vi "temp_probe_calibrator.vi"() -> ()   [LabVIEW 2010]
uses:
  <vilib>/Instr/_visa.llb/VISA Configure Serial Port (Instr).vi
  <vilib>/Utility/file.llb/Write To Spreadsheet File (string).vi
  <vilib>/Analysis/NI_AALBase.lvlib
  <vilib>/Analysis/NI_AALPro.lvlib
panel:
  out "estimatedTemps":dbl[](array[numeric]) format="%.3g"
  out "XY Graph":T1(graph)
  in  "Path":path=path "C:/Users/OA-user/Documents/OAlab/data"
  in  "fileName":string="tempProbe_cal_data_"
  out "CalOutput":string[][](array[string])
  in  "RefText":string="fluke_1523_#1085081"
  in  "headers":string[](array[string])=["location", "probeType", "channel", "Ohm->Temp", "date", "reference"]
  in  "labels":string[][](array[string])=[["cell", "TJ36-44004-1/8"], ["acidBottle", "TJ36-44004-1/8"], ["burrette1", "SA1-TH-44004-40-T"], ["burrette2", "SA1-TH-44004-40-T"], ["room", "unknown"]]
  out "currentSet":dbl format="%.3g"
  out "currentPoint":i32=20
  out "numPoints":i32=20
  out "rawOhmsAll":dbl[][](array[numeric])
  out "flukeTempsAll":dbl[](array[numeric]) format="%.3g"
  out "FlukeTempAvg":dbl format="%.3g"
  in  "chillTemps":dbl[](array[numeric])
  out "Waveform Chart":dbl(graph)
  out "currentTime":timestamp format="%<%X>T"
  out "lastRead":timestamp format="%<%X>T"
  in  "nextRead":timestamp format="%<%X>T"
  in  "Neslab Port IN":refnum<visa-resource-name>="COM12"
  in  "minutes@temp":dbl=20.0
  out "rawOhm":dbl[](array[numeric])
  out "FlukeTemp":dbl format="%.3g"
  in  "stop":bool
  in  "Agilent Settings":T2={"Agilent COM Port"="", "Probe Channels (csv)"="103,104,105,106,107", "Number of Readings"=10}
  in  "Fluke Settings":T3={"COM Port"="COM13", "Baud Rate"=9600, "Data Bit"=8, "Parity"=0, "Bytes to Read"=7}
  out "error out":errorcluster
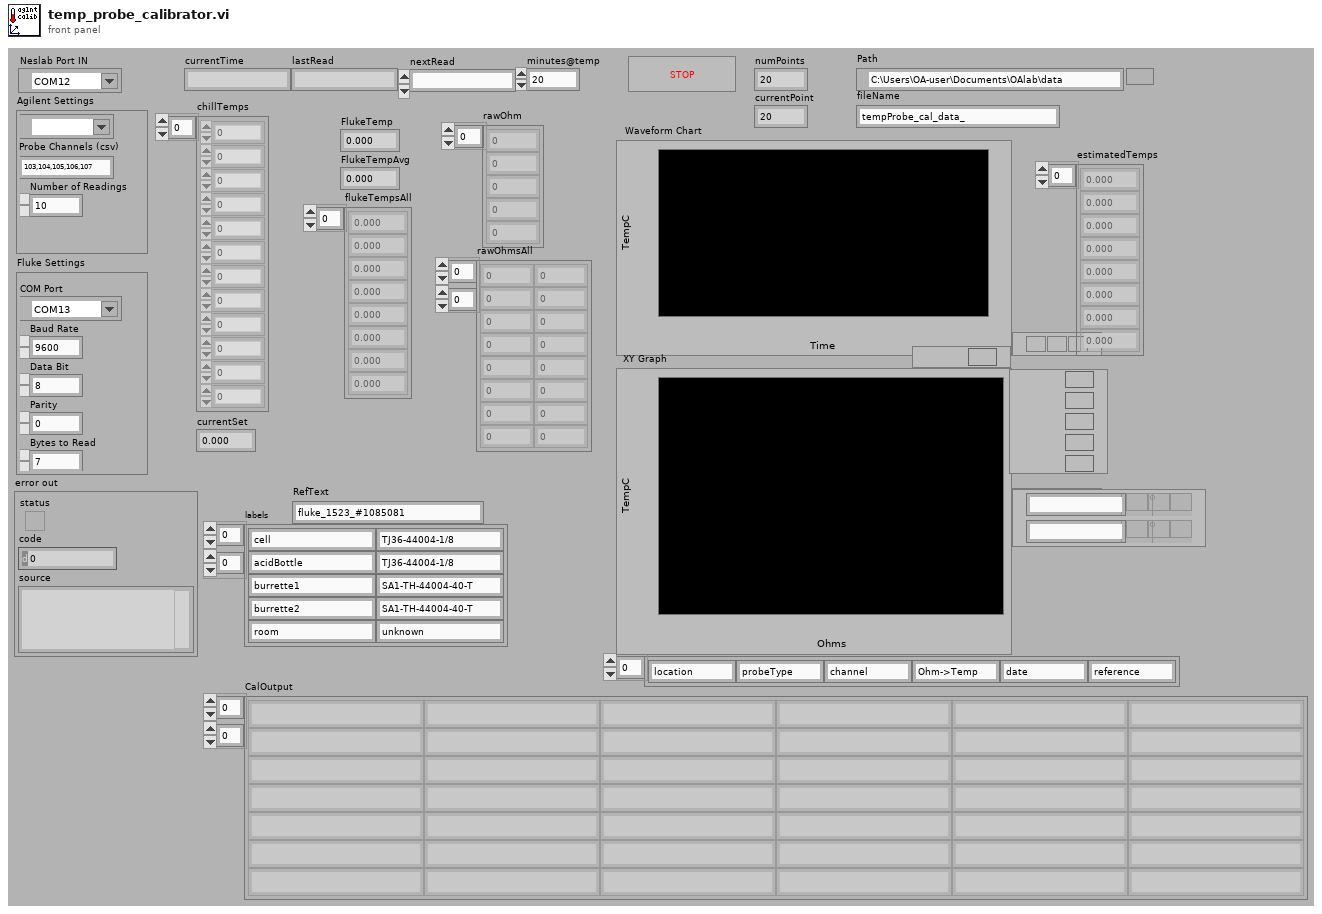
[diagram p1: front panel]
types:
  T1 = cluster{"flukeTempsAll":dbl[], "rawOhmsAll":dbl[]}[]
  T2 = cluster{"Agilent COM Port":refnum<visa-resource-name>, "Probe Channels (csv)":string, "Number of Readings":i32}
  T3 = cluster{"COM Port":refnum<visa-resource-name>, "Baud Rate":u32, "Data Bit":i8, "Parity":i8, "Bytes to Read":u32}
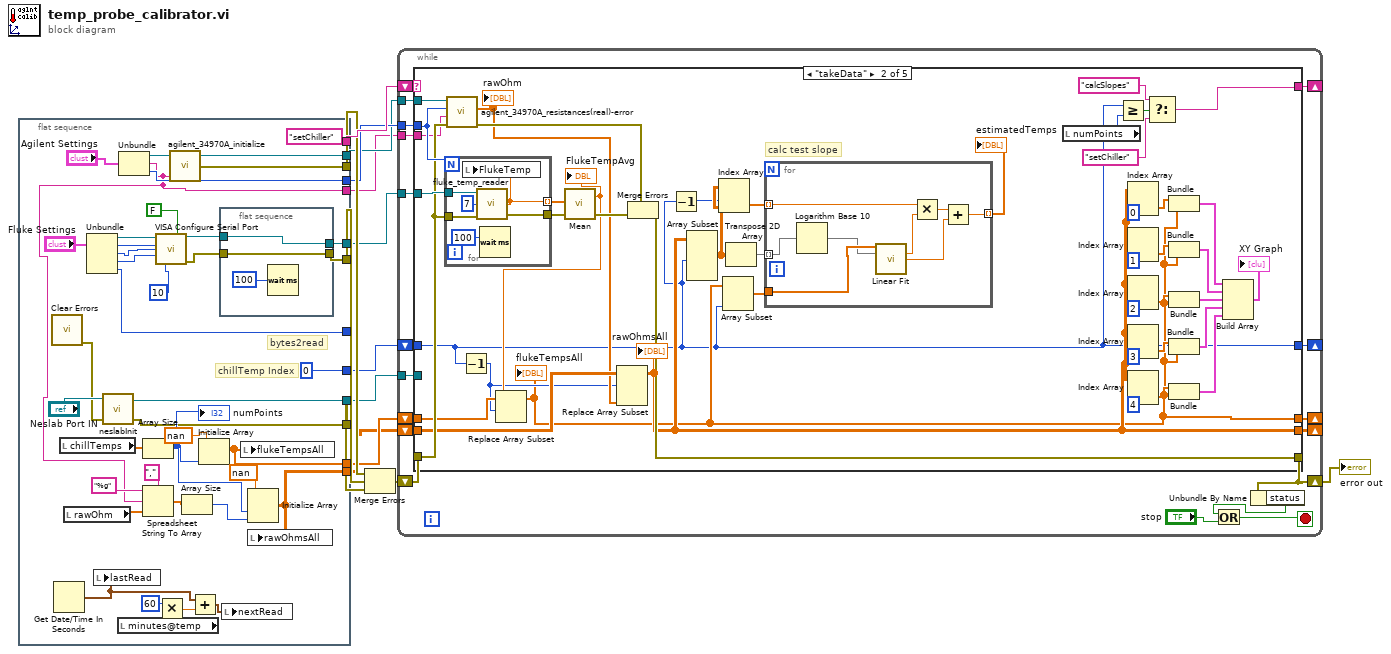
[diagram p0: block diagram]
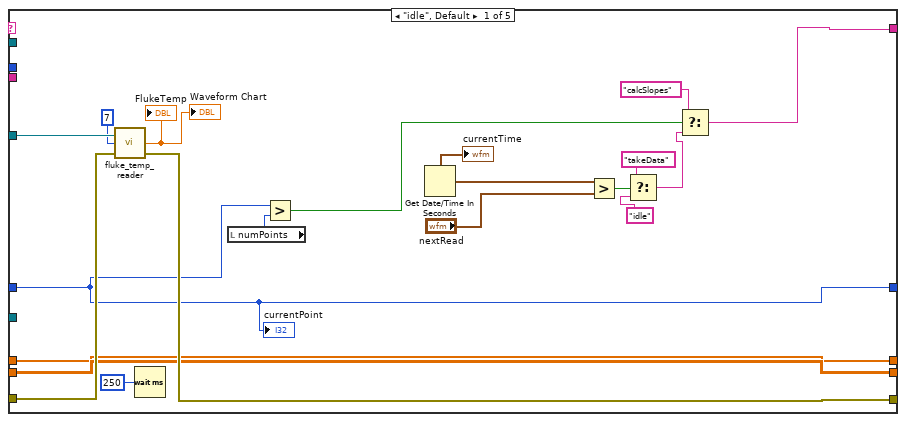
[diagram p2: hidden frame]
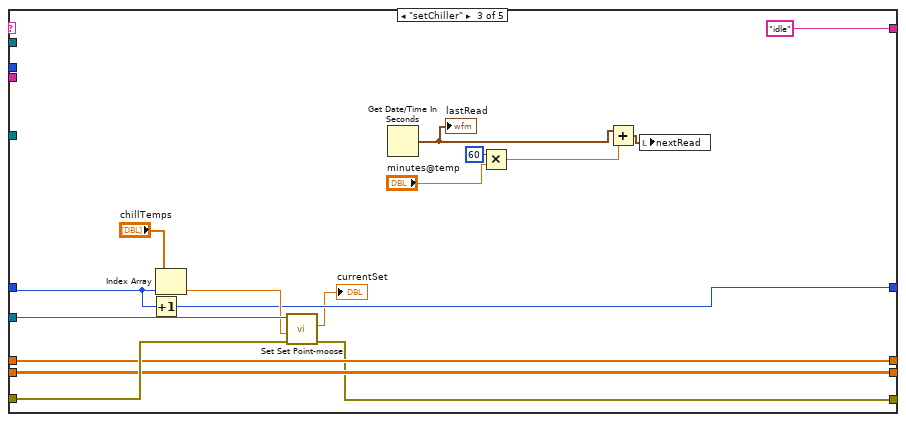
[diagram p3: hidden frame]
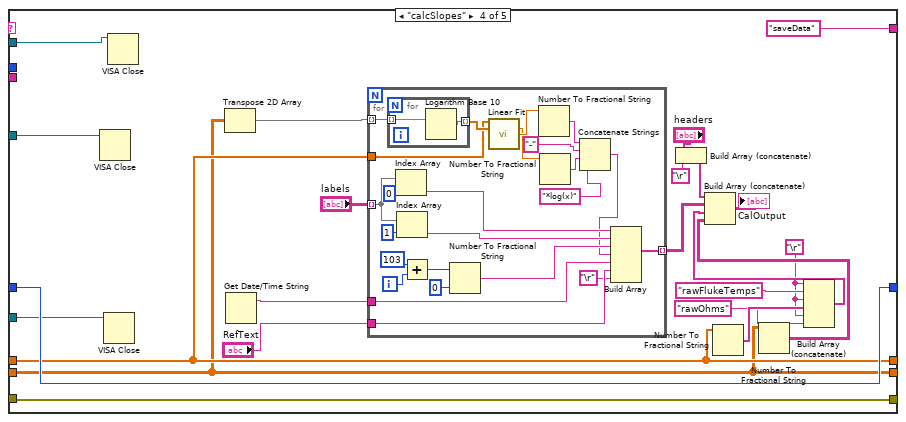
[diagram p4: hidden frame]
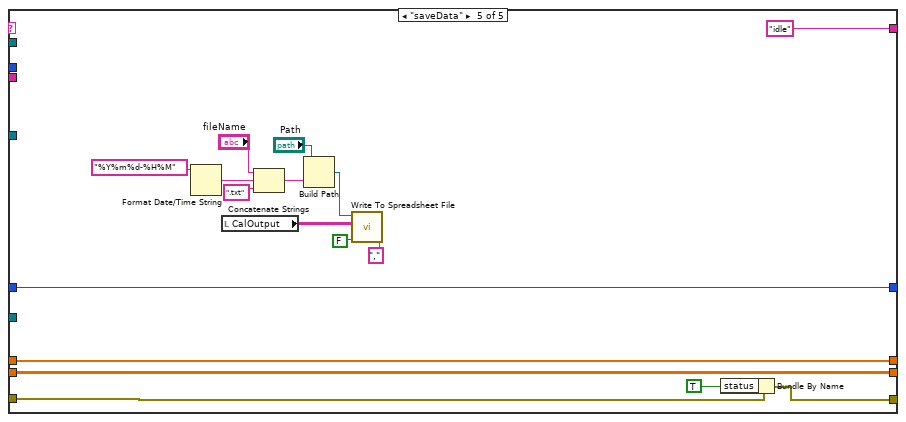
[diagram p5: hidden frame]
diagram:
  n1 = flat-sequence {
    tunnel: [w52] -> w9
    tunnel: [w50] -> w12
    tunnel: [w48] -> w5
    tunnel: [w47] -> w13
    tunnel: [w41] -> _
    tunnel: [w38] -> w6
    tunnel: [w30] -> w1
    tunnel: [w16] -> w11
    tunnel: ["setChiller"] -> w14
    tunnel: [w17] -> w8
    tunnel: [0] -> w7
    tunnel: [w24] -> w4
    tunnel: [w23] -> w3
    frame #0 {
      # "chillTemp Index"
      # "bytes2read"
      n2 = call <vilib>:"Clear Errors.vi"() -> ("error out"=w15:errorcluster)  [unwired: 7 in]
      n3 = Get Date/Time In Seconds() -> (seconds since 1Jan1904=w36:timestamp)
      n4 = local read "chillTemps"() -> (w29:dbl[])
      n5 = local read "rawOhm"() -> (w26:dbl[])
      n6 = Unbundle("Fluke Settings") -> ("COM Port"=w45:refnum<visa-resource-name>, "Baud Rate"=w44:u32, "Data Bit"=w43:i8, "Parity"=w42:i8, "Bytes to Read"=w41:u32)
      n7 = local write "lastRead"(w36) -> ()
      n8 = call "neslabInit.vi"("error in (no error)"=w15, "COM Port"="Neslab Port IN") -> ("error out"=w16:errorcluster, "COM Port Out"=w17:refnum<visa-resource-name>)  [unwired: 1 in, 1 out]
      n9 = local read "minutes@temp"() -> (w19:dbl)
      n10 = Unbundle("Agilent Settings") -> ("Agilent COM Port"=w39:refnum<visa-resource-name>, "Probe Channels (csv)"=w30:string, "Number of Readings"=w38:i32)
      n11 = Array Size(array=w29) -> (size(s)=w22:i32)
      "numPoints" <- w22
      n12 = Spreadsheet String To Array(delimiter (Tab)=",", format string="%g", spreadsheet string=w30, array type (2D Dbl)=w26) -> (array=w33:dbl[])
      n13 = call-poly "VISA Configure Serial Port"("VISA resource name"=w45, "Enable Termination\nChar (T)"=FALSE, "baud rate (9600)"=w44, "data bits (8)"=w43, "parity (0:none)"=w42, "stop bits (10: 1 bit)"=10) -> ("VISA resource name out"=w51:refnum<visa-resource-name>, "error out"=w49:errorcluster)  [unwired: 8 in]
      n14 = Multiply(x=60, y=w19) -> (x*y=w20:dbl)
      n15 = call "agilent_34970A_initialize.vi"("resistance channels (csv)"=w30, "Agilent 34970A Port"=w39) -> ("34970A Error Out"=w47:errorcluster, "34970A Port Out"=w48:refnum<visa-resource-name>)  [unwired: 1 in, 1 out]
      n16 = Array Size(array=w33) -> (size(s)=w25:i32)
      n17 = Add(x=w36, y=w20) -> (x+y=w35:timestamp)
      n18 = Initialize Array(nan ("FlukeTempAvg"), w22) -> (w24:dbl[])
      n19 = flat-sequence {
        tunnel: [w56] -> w52
        tunnel: w51 -> [w56]
        tunnel: [w55] -> w50
        tunnel: w49 -> [w55]
        frame #0 {
          n20 = Wait (ms)(milliseconds to wait=100) -> ()  [unwired: 1 out]
        }
      }
      n21 = local write "nextRead"(w35) -> ()
      n22 = local write "flukeTempsAll"(w24) -> ()
      n23 = Initialize Array(nan ("FlukeTempAvg"), w22, w25) -> (w23:dbl[][])
      n24 = local write "rawOhmsAll"(w23) -> ()
    }
  }
  n25 = Merge Errors(w13, w12, w11) -> (w10:errorcluster)
  n26 = while {
    shift-right: [w60] -> w2
    shift-left: w10 -> [w74]
    tunnel: w9 -> [w73]
    tunnel: w8 -> [w72]
    shift-right: [w70] -> _
    shift-left: w7 -> [w71]
    shift-right: [w69] -> _
    shift-left: w14 -> [w75]
    tunnel: w6 -> [w68]
    tunnel: w5 -> [w67]
    shift-right: [w64] -> _
    shift-left: w4 -> [w66]
    shift-right: [w63] -> _
    shift-left: w3 -> [w65]
    tunnel: w1 -> [w58]
    stop <- w61 stop-if-true
    n27 = case shown="\"takeData\"" w75 {
      tunnel: w74 -> [w93 w134 w167 w189 w220]
      tunnel: w73 -> [w92 w137 _ w186 _]
      tunnel: w72 -> [_ _ w168 w187 _]
      tunnel: w71 -> [w76 w95 w164 w190 w231]
      tunnel: [w76 w95 w156 w190 w231] -> w70
      tunnel: [w88 w127 w154 w189 w219] -> w60
      tunnel: [w78 w121 "idle" "saveData" "idle"] -> w69
      tunnel: w68 -> [_ w136 _ _ _]
      tunnel: w67 -> [_ w138 _ w188 _]
      tunnel: w66 -> [w86 w130 w160 w178 w232]
      tunnel: w65 -> [w87 w129 w161 w175 w233]
      tunnel: [w86 w97 w160 w178 w232] -> w64
      tunnel: [w87 w106 w161 w175 w233] -> w63
      tunnel: w58 -> [_ w126 _ _ _]
      frame "idle", Default {
        n28 = call "fluke_temp_reader.vi"("error in (no error)"=w93, "Bytes to Read"=7, "COM Port In"=w92) -> ("error out"=w88:errorcluster, "Temp"=→"FlukeTemp" →"Waveform Chart":dbl)  [unwired: 1 out]
        n29 = Wait (ms)(milliseconds to wait=250) -> ()  [unwired: 1 out]
        n30 = local read "numPoints"() -> (w82:i32)
        n31 = Greater?(x=w76, y=w82) -> (0:w80:bool)
        n32 = Get Date/Time In Seconds() -> (seconds since 1Jan1904=w90:timestamp)
        "currentTime" <- w90
        n33 = Greater?(x=w90, y="nextRead") -> (0:w84:bool)
        n34 = Select(t="takeData", s=w84, f="idle") -> (s? t:f=w81:string)
        n35 = Select(t="calcSlopes", s=w80, f=w81) -> (s? t:f=w78:string)
        "currentPoint" <- w76
      }
      frame "takeData" {
        # "calc test slope"
        n36 = for {
          N: w136 -> [_]
          tunnel: w137 -> [w152]
          tunnel: w134 -> [w151]
          tunnel: [w150] -> w135 mode=indexing
          tunnel: [w149] -> w133
          n37 = call "fluke_temp_reader.vi"("error in (no error)"=w151, "Bytes to Read"=7, "COM Port In"=w152) -> ("error out"=w149:errorcluster, "Temp"=w150:dbl)  [unwired: 1 out]
          n38 = local write "FlukeTemp"(w150) -> ()
          n39 = Wait (ms)(milliseconds to wait=100) -> ()  [unwired: 1 out]
        }
        n40 = call "agilent_34970A_resistances(real)-error.vi"("error in (no error)"=w134, "Channels"=w126, "Readings"=w136, "Agilent Port In"=w138) -> ("error out"=w132:errorcluster, "Resistances"=w128:dbl[])  [unwired: 2 out]
        "rawOhm" <- w128
        n41 = Decrement(x=w95) -> (x-1=w109:i32)
        n42 = call <vilib>:"Mean.vi"("X"=w135) -> ("mean"=w131:dbl)  [unwired: 1 out]
        "FlukeTempAvg" <- w131
        n43 = Replace Array Subset(array=w130, new element=w131, index=w109) -> (w97:dbl[])
        "flukeTempsAll" <- w97
        n44 = Replace Array Subset(array=w129, new element=w128, index (row)=w109) -> (w106:dbl[][])  [unwired: 1 in]
        "rawOhmsAll" <- w106
        n45 = Merge Errors(w132, w133) -> (w127:errorcluster)
        n46 = Decrement(x=w95) -> (x-1=w96:i32)
        n47 = Array Subset(array=w106, length (row)=w95) -> (w104:dbl[][])  [unwired: 3 in]
        n48 = Index Array(array=w104, index (row)=w96) -> (element=w103:dbl[])  [unwired: 1 in]
        n49 = Array Subset(array=w97, length=w95) -> (w107:dbl[])  [unwired: 1 in]
        n50 = Transpose 2D Array(2D array=w104) -> (transposed array=w108:dbl[][])
        n51 = for {
          tunnel: w108 -> [w142] mode=indexing
          tunnel: w107 -> [w141]
          tunnel: [w143] -> w105 mode=indexing
          tunnel: w103 -> [w139] mode=indexing
          n52 = Logarithm Base 10(1:w142) -> (0:w140:dbl[])
          n53 = call <vilib>:"Linear Fit.vi"("Y"=w141, "X"=w140) -> ("slope"=w146:dbl, "intercept"=w144:dbl)  [unwired: 9 in, 3 out]
          n54 = Multiply(x=w139, y=w146) -> (x*y=w145:dbl)
          n55 = Add(x=w145, y=w144) -> (x+y=w143:dbl)
        }
        "estimatedTemps" <- w105
        n56 = local read "numPoints"() -> (w125:i32)
        n57 = Greater Or Equal?(x=w95, y=w125) -> (x >= y?=w124:bool)
        n58 = Index Array(array=w106, index (col)=0) -> (element=w102:dbl[])  [unwired: 1 in]
        n59 = Index Array(array=w106, index (col)=1) -> (element=w101:dbl[])  [unwired: 1 in]
        n60 = Index Array(array=w106, index (col)=2) -> (element=w100:dbl[])  [unwired: 1 in]
        n61 = Index Array(array=w106, index (col)=3) -> (element=w99:dbl[])  [unwired: 1 in]
        n62 = Index Array(array=w106, index (col)=4) -> (element=w98:dbl[])  [unwired: 1 in]
        n63 = Select(t="calcSlopes", s=w124, f="setChiller") -> (s? t:f=w121:string)
        n64 = Bundle(w102, w97) -> (w115:cluster{dbl[], dbl[]})  [unwired: 1 in]
        n65 = Bundle(w101, w97) -> (w113:cluster{dbl[], dbl[]})  [unwired: 1 in]
        n66 = Bundle(w100, w97) -> (w114:cluster{dbl[], dbl[]})  [unwired: 1 in]
        n67 = Bundle(w99, w97) -> (w112:cluster{dbl[], dbl[]})  [unwired: 1 in]
        n68 = Bundle(w98, w97) -> (w111:cluster{dbl[], dbl[]})  [unwired: 1 in]
        n69 = Build Array(w115, w113, w114, w112, w111) -> (→"XY Graph":cluster{dbl[], dbl[]}[])
      }
      frame "setChiller" {
        n70 = Increment(x=w164) -> (x+1=w156:i32)
        n71 = Index Array(array="chillTemps", index=w164) -> (element=w165:dbl)
        n72 = call "Set Set Point-moose.vi"("COM Port IN"=w168, "Numerical\nSet Value"=w165, "error in\n(no error)"=w167) -> ("Numeric\nReading Value"=→"currentSet":dbl, "error out"=w154:errorcluster)  [unwired: 3 in, 2 out]
        n73 = Get Date/Time In Seconds() -> (seconds since 1Jan1904=w159:timestamp)
        "lastRead" <- w159
        n74 = Multiply(x=60, y="minutes@temp") -> (x*y=w157:dbl)
        n75 = Add(x=w159, y=w157) -> (x+y=w162:timestamp)
        n76 = local write "nextRead"(w162) -> ()
      }
      frame "calcSlopes" {
        w172 = "\r"
        n77 = VISA Close(VISA resource name=w186) -> ()  [unwired: 1 in, 1 out]
        n78 = VISA Close(VISA resource name=w187) -> ()  [unwired: 1 in, 1 out]
        n79 = VISA Close(VISA resource name=w188) -> ()  [unwired: 1 in, 1 out]
        n80 = Transpose 2D Array(2D array=w175) -> (transposed array=w185:dbl[][])
        n81 = Get Date/Time String() -> (date string=w183:string)  [unwired: 3 in, 1 out]
        n82 = for {
          tunnel: w185 -> [w215] mode=indexing
          tunnel: w178 -> [w194]
          tunnel: "labels" -> [w213] mode=indexing
          tunnel: w183 -> [w203]
          tunnel: "RefText" -> [w202]
          tunnel: [w201] -> w181 mode=indexing
          i -> [w211]
          n83 = for {
            tunnel: w215 -> [w217] mode=indexing
            tunnel: [w216] -> w195 mode=indexing
            n84 = Logarithm Base 10(1:w217) -> (0:w216:dbl)
          }
          n85 = Index Array(array=w213, index=0) -> (element=w207:string)
          n86 = Index Array(array=w213, index=1) -> (element=w206:string)
          n87 = Add(x=103, y=w211) -> (x+y=w209:i32)
          n88 = Number To Fractional String(number=w209, precision (6)=0) -> (F-format string=w205:string)  [unwired: 2 in]
          n89 = call <vilib>:"Linear Fit.vi"("Y"=w194, "X"=w195) -> ("slope"=w192:dbl, "intercept"=w193:dbl)  [unwired: 9 in, 3 out]
          n90 = Number To Fractional String(number=w193) -> (F-format string=w208:string)  [unwired: 3 in]
          n91 = Number To Fractional String(number=w192) -> (F-format string=w199:string)  [unwired: 3 in]
          n92 = Concatenate Strings(w208, "-", w199, "*log(x)") -> (w204:string)
          n93 = Build Array(w207, w206, w205, w204, w203, w202, "\r") -> (w201:string[])
        }
        n94 = Build Array (concatenate)("headers", "\r") -> (w169:string[])
        n95 = Number To Fractional String(number=w178) -> (F-format string=w177:string[])  [unwired: 3 in]
        n96 = Number To Fractional String(number=w175) -> (F-format string=w173:string[][])  [unwired: 3 in]
        n97 = Build Array (concatenate)(w172, "rawFlukeTemps", w172, w177, w172, "rawOhms") -> (w174:string[])
        n98 = Build Array (concatenate)(w169, w181, w174, w173) -> (→"CalOutput":string[][])
      }
      frame "saveData" {
        n99 = Format Date/Time String(time format string (%c)="%Y%m%d-%H%M") -> (date/time string=w222:string)  [unwired: 2 in]
        n100 = local read "CalOutput"() -> (w221:string[][])
        n101 = Concatenate Strings("fileName", w222, ".txt") -> (w228:string)
        n102 = Build Path(base path="Path", name or relative path=w228) -> (appended path=w226:path)
        n103 = call-poly <vilib>:"Write To Spreadsheet File.vi"("delimiter (\\t)"=",", "append to file? (new file:F)"=FALSE, "2D data"=w221, "file path (dialog if empty)"=w226) -> ()  [unwired: 4 in, 1 out]
        n104 = Bundle By Name(cluster=w220, "status"=TRUE) -> (w219:errorcluster)
      }
    }
    n105 = Unbundle By Name(w60) -> ("status"=w59:bool)
    n106 = Or(x=w59, y="stop") -> (x .or. y?=w61:bool)
  }
  "error out" <- w2
